vi "Manage Dirty Field ID List.vi"(10 "Operation":enum16{"Mark", "Retrieve/Clear", "Mark Flags"}(ring), 11 "Field ID":T1) -> (2 "Field IDs Flags":T1[](array[typedef]), 3 "Field IDs":T1[](array[typedef]))   [LabVIEW 2017]
doc: "Maintain the list of variables whose value has been modified and not yet transmitted to other clients."
uses:
  <vilib>/Rock Robotics/Network Tables/Field ID.ctl
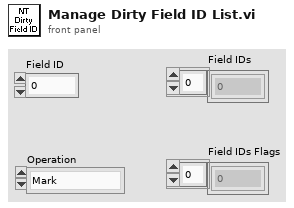
[diagram p1: front panel]
types:
  T1 = typedef "Field ID.ctl" = i32
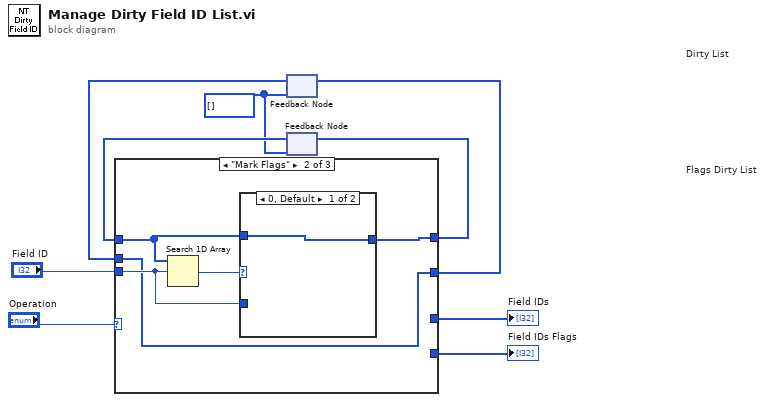
[diagram p0: block diagram]
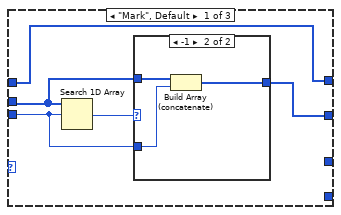
[diagram p2: hidden frame]
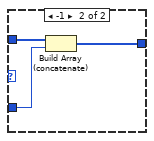
[diagram p4: hidden frame]
diagram:
  w2 = T1[] [] ("Field IDs")
  n1 = feedback #1 "Dirty List"(w2) -> (w6:T1[])
  n2 = feedback #2 "Flags Dirty List"(w2) -> (w4:T1[])
  n3 = case shown="\"Mark Flags\"" "Operation" {
    tunnel: w6 -> [w13 w21 w29]
    tunnel: [w14 w21 _] -> w5
    tunnel: "Field ID" -> [w12 w23 _]
    tunnel: [_ _ w29] -> w7
    tunnel: w4 -> [w10 w20 w28]
    tunnel: [w10 w19 _] -> w3
    tunnel: [_ _ w28] -> w1
    frame "Mark", Default {
      n4 = Search 1D Array(1D array=w13, element=w12) -> (index of element=w11:i32)  [unwired: 1 in]
      n5 = case shown="-1" w11 {
        tunnel: w13 -> [w15 w18]
        tunnel: w12 -> [_ w17]
        tunnel: [w15 w16] -> w14
        frame 0, Default {
        }
        frame -1 {
          n6 = Build Array (concatenate)(w18, w17) -> (w16:T1[])
        }
      }
    }
    frame "Mark Flags" {
      n7 = Search 1D Array(1D array=w20, element=w23) -> (index of element=w22:i32)  [unwired: 1 in]
      n8 = case shown="0, Default" w22 {
        tunnel: w20 -> [w24 w27]
        tunnel: w23 -> [_ w26]
        tunnel: [w24 w25] -> w19
        frame 0, Default {
        }
        frame -1 {
          n9 = Build Array (concatenate)(w27, w26) -> (w25:T1[])
        }
      }
    }
    frame "Retrieve/Clear" {
    }
  }
  "Field IDs" <- w7
  "Field IDs Flags" <- w1
  n10 = feedback-in #1(w5) -> ()
  n11 = feedback-in #2(w3) -> ()
